vi "XPS hardware acquire.vi"(8 "error in (no error)":errorcluster, 11 "Object in":refnum<class "NewportXPS.lvclass">) -> (0 "error out":errorcluster, 3 "Object out":refnum<class "NewportXPS.lvclass">)   [LabVIEW 2020, in "NewportXPS.lvclass"]
uses:
  NewportXPS.lvclass
  XPS Acquire FGV.ctl
  stop FGV control.ctl
  NewportXPS.lvclass/NewportXPS.ctl
  DriverMsg.ctl
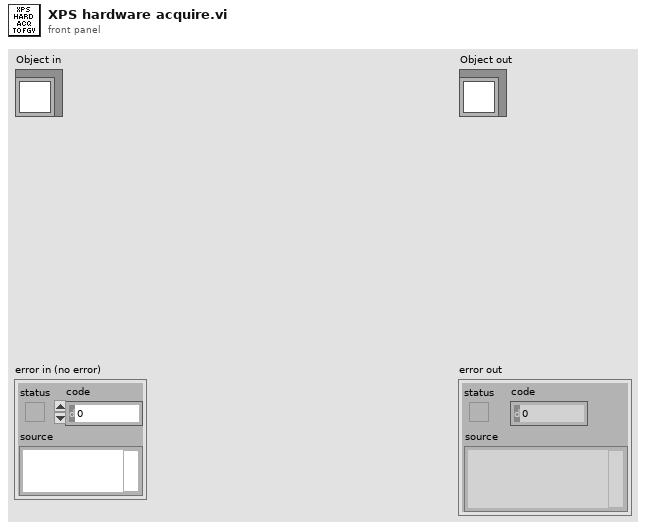
[diagram p1: front panel]
types:
  T1 = typedef "stop FGV control.ctl" = enum16{"Clear", "Write", "Read"}
  T2 = typedef "XPS Acquire FGV.ctl" = cluster{"busy":bool, "positions":dbl[]}
  T3 = cluster{"Axis 1":cluster{"Value":dbl, "Min":dbl, "Max":dbl, "StepSize":dbl, "Tolerance":dbl, "ValueActual":dbl}, "Axis 2":cluster{"Value":dbl, "Min":dbl, "Max":dbl, "StepSize":dbl, "Tolerance":dbl, "ValueActual":dbl}, "Axis 3":cluster{"Value":dbl, "Min":dbl, "Max":dbl, "StepSize":dbl, "Tolerance":dbl, "ValueActual":dbl}, "Axis 4":cluster{"Value":dbl, "Min":dbl, "Max":dbl, "StepSize":dbl, "Tolerance":dbl, "ValueActual":dbl}, "Axis 5":cluster{"Value":dbl, "Min":dbl, "Max":dbl, "StepSize":dbl, "Tolerance":dbl, "ValueActual":dbl}, "Axis 6":cluster{"Value":dbl, "Min":dbl, "Max":dbl, "StepSize":dbl, "Tolerance":dbl, "ValueActual":dbl}}
  T4 = cluster{"connection TCP":refnum<k5>, "LogTo File":bool, "Log File refnum":refnum<file>, "no error if error log":bool}
  T5 = cluster{"Axis 1":string, "Axis 2":string, "Axis 3":string, "Axis 4":string, "Axis 5":string, "Axis 6":string}
  T6 = typedef "DriverMsg.ctl" = cluster{"Command":string, "Args":string[]}
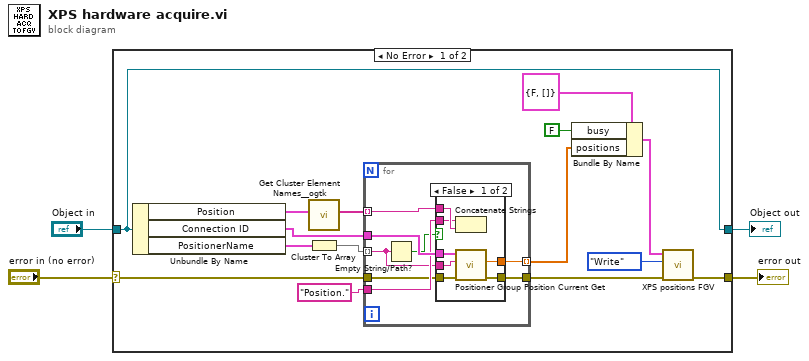
[diagram p0: block diagram]
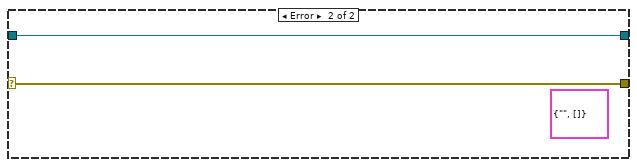
[diagram p3: hidden frame]
diagram:
  n1 = case shown="No Error" "error in (no error)" {
    selector: "error in (no error)" -> [w12 w37]
    tunnel: [w6 w37] -> w1
    tunnel: [w13 w36] -> w4
    tunnel: "Object in" -> [w13 w36]
    frame No Error {
      n2 = Unbundle By Name(w13) -> ("Position"=w15:T3, "Connection ID"=w18:T4, "PositionerName"=w17:T5)
      n3 = call "Get Cluster Element Names__ogtk.vi"("Cluster"=w15) -> ("Element Names"=w14:string[])  [unwired: 9 in, 1 out]
      n4 = Cluster To Array(cluster=w17) -> (array=w16:string[])
      n5 = for {
        tunnel: "Position." ("command or variable name") -> [w24]
        tunnel: w18 -> [w27]
        tunnel: [w26] -> w7
        tunnel: w16 -> [w22] mode=indexing
        tunnel: w14 -> [w25] mode=indexing
        tunnel: w12 -> [w23]
        tunnel: [w21] -> w9 mode=indexing
        n6 = Empty String/Path?(string/path=w22) -> (empty?=w20:bool)
        n7 = case shown="False" w20 {
          tunnel: w27 -> [w34 _]
          tunnel: [w29 w35] -> w26
          tunnel: w25 -> [w33 _]
          tunnel: w24 -> [w32 _]
          tunnel: w23 -> [w31 w35]
          tunnel: w22 -> [w30 _]
          tunnel: [w28 _] -> w21
          frame False {
            n8 = Concatenate Strings(w32, w33) -> ()  [unwired: 1 out]
            n9 = call "Positioner Group Position Current Get.vi"("error in (no error)"=w31, "Positioner Name (250 c max)"=w30, "connection ID in"=w34) -> ("error out"=w29:errorcluster, "Current position (units)"=w28:dbl)  [unwired: 5 in, 2 out]
          }
          frame True {
          }
        }
      }
      n10 = Bundle By Name(cluster=T2 {"busy"=FALSE, "positions"=[]} ("Acq Data in"), "busy"=FALSE, "positions"=w9) -> (w10:T2)
      n11 = call "XPS positions FGV.vi"("error in"=w7, "Function"=stop_FGV_control."Write", "Acq Data in"=w10) -> ("error out"=w6:errorcluster)  [unwired: 7 in, 1 out]
    }
    frame Error {
      (unwired) T6 {"Command"="", "Args"=[]} ("Msg out")
    }
  }
  "error out" <- w1
  "Object out" <- w4
